vi "读取数值.vi"(8 "error in (no error)":errorcluster, 10 "Slave ID":u8=1, 11 "MB session in":refnum<class "MB_Master.lvclass">) -> (0 "error out":errorcluster, 2 "读取值":T1, 3 "MB session out":refnum<class "MB_Master.lvclass">)   [LabVIEW 2016, in "流量计集成.lvlib" / "WL1A1明渠流量计.lvlib"]
uses:
  <vilib>/Plasmionique/MB Master/MB_Master/MB_Master.lvclass
  <vilib>/Plasmionique/MB Master/MB Master.lvlib
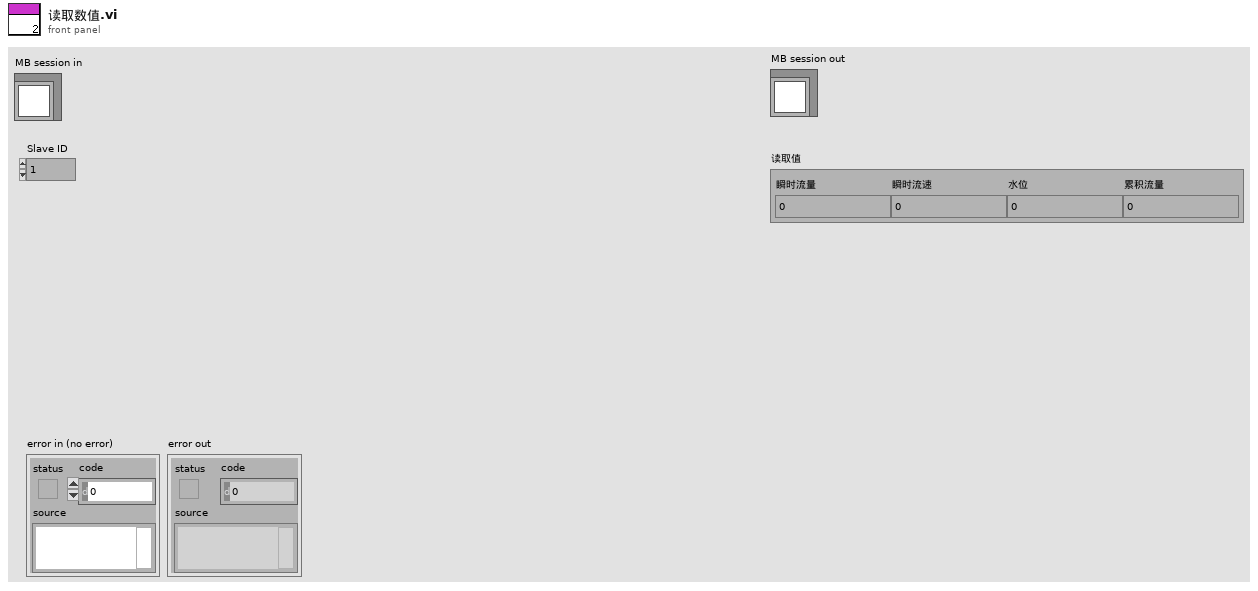
[diagram p1: front panel]
types:
  T1 = typedef "流量计集成.lvlib/博意达流量计.lvlib/读取值.ctl" = cluster{"瞬时流量":sgl, "瞬时流速":sgl, "水位":sgl, "累积流量":sgl}
  T2 = cluster{"瞬时流量L/s":dbl, "瞬时流量m3/h":dbl, "累计流量m3":dbl, "液位m":dbl, "I1":dbl, "I2":dbl, "I3":dbl, "I4":dbl}
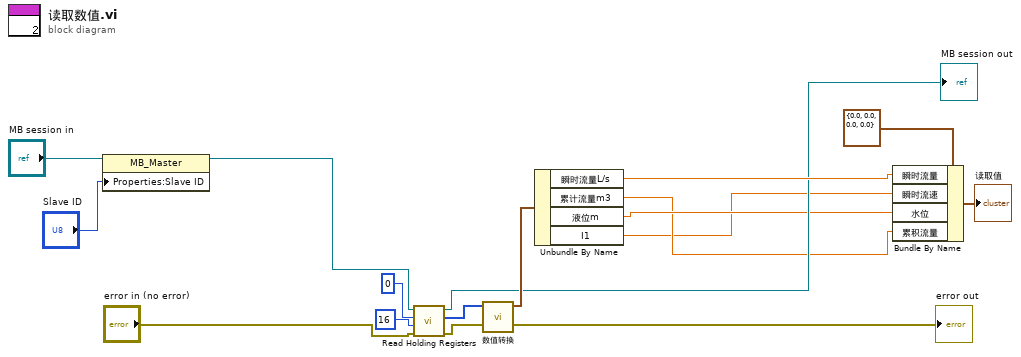
[diagram p0: block diagram]
diagram:
  n1 = property class="MB_Master"(reference="MB session in", "Properties:Slave ID"="Slave ID") -> (reference out=w9:refnum<class "MB_Master.lvclass">)  [unwired: 1 in, 1 out]
  n2 = call <vilib>:"Read Holding Registers.vi"("error in (no error)"="error in (no error)", "quantity"=u16 16, "starting address"=u16 0, "MB session in"=w9) -> ("error out"=→"error out":errorcluster, "Registers"=w10:u16[], "MB session out"=→"MB session out":refnum<class "MB_Master.lvclass">)  [unwired: 5 in]
  n3 = call "数值转换.vi"("数组"=w10) -> ("显示值"=w7:T2)  [unwired: 10 in]
  n4 = Unbundle By Name(w7) -> ("瞬时流量L/s"=w6:dbl, "累计流量m3"=w2:dbl, "液位m"=w3:dbl, "I1"=w1:dbl)
  n5 = Bundle By Name(cluster=T1 {"瞬时流量"=0.0, "瞬时流速"=0.0, "水位"=0.0, "累积流量"=0.0} ("读取值"), "瞬时流量"=w6, "瞬时流速"=w1, "水位"=w3, "累积流量"=w2) -> (→"读取值":T1)
